vi "RDS Serial Frame Write.vi"(8 "error in (no error)":errorcluster, 9 "Time Stamp":timestamp, 10 "Serial String":string, 11 "RDS Serial Frame in":refnum<class "RDS Serial Frame.lvclass">) -> (0 "error out":errorcluster, 3 "RDS Serial Frame out":refnum<class "RDS Serial Frame.lvclass">)   [LabVIEW 2015, in "RDS Serial Handler.lvlib" / "RDS Serial Frame.lvclass"]
uses:
  RDS Serial Frame.lvclass
  RDS Serial Frame.lvclass/RDS Serial Frame.ctl
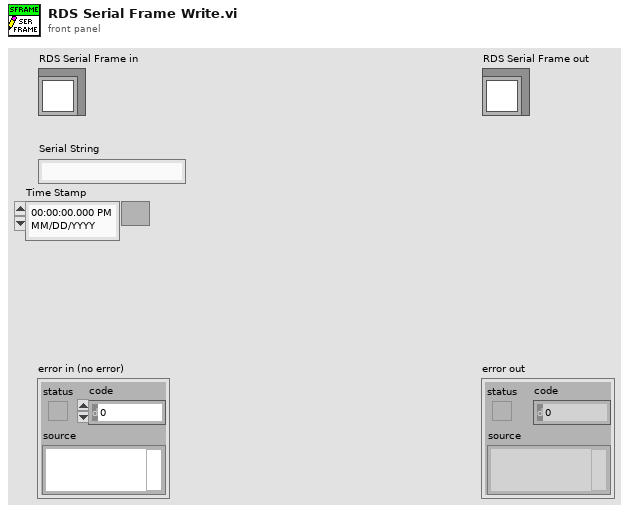
[diagram p1: front panel]
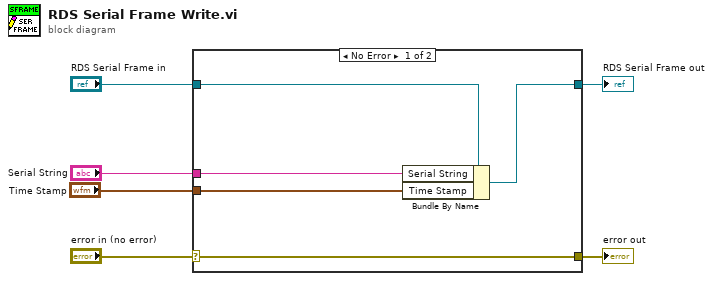
[diagram p0: block diagram]
diagram:
  n1 = case shown="No Error" "error in (no error)" {
    selector: "error in (no error)" -> [w11 w12]
    tunnel: [w11 w12] -> w5
    tunnel: [w9 w13] -> w3
    tunnel: "RDS Serial Frame in" -> [w10 w13]
    tunnel: "Serial String" -> [w8 _]
    tunnel: "Time Stamp" -> [w7 _]
    frame No Error {
      n2 = Bundle By Name(cluster=w10, "Serial String"=w8, "Time Stamp"=w7) -> (w9:refnum<class "RDS Serial Frame.lvclass">)
    }
    frame Error {
    }
  }
  "error out" <- w5
  "RDS Serial Frame out" <- w3
